vi "Material-Automation-LaunchWirebirdLabsWebsite.vi"(0 "Site to Launch":T1, 11 "error in":errorcluster) -> (15 "error out":errorcluster)   [LabVIEW 2013]
uses:
  Material-Automation-Website.ctl
panel:
  # "Inputs"
  # "Outputs"
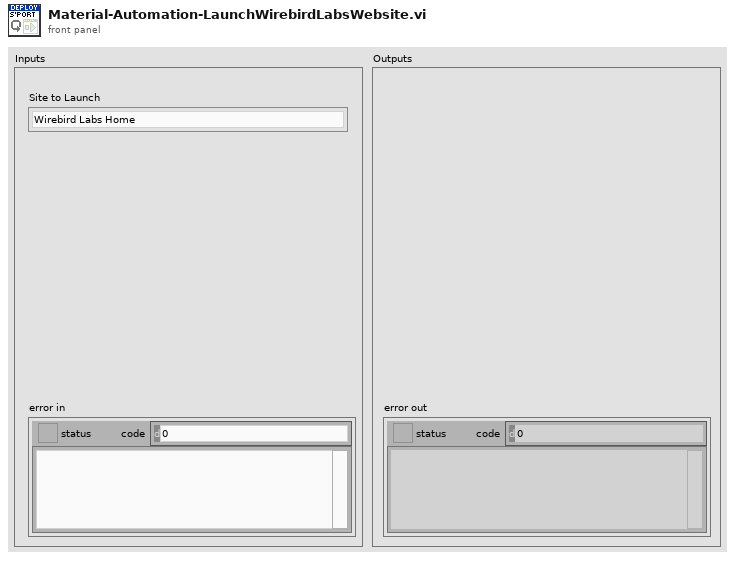
[diagram p1: front panel]
types:
  T1 = typedef "Material-Automation-Website.ctl" = enum16{"Wirebird Labs Home", "Wirebird Labs Support Home", "Wirebird Labs Licensing", "Wirebird Labs Idea Exchange", "Wirebird Labs Report a Bug", "Wirebird Labs Services Status", "Contact Wirebird Labs", "Deploy Documentation", "Deploy Credits", "Deploy Marketing", "Deploy Feature Matrix", "Deploy Purchase", "Deploy Deployment Servers"}
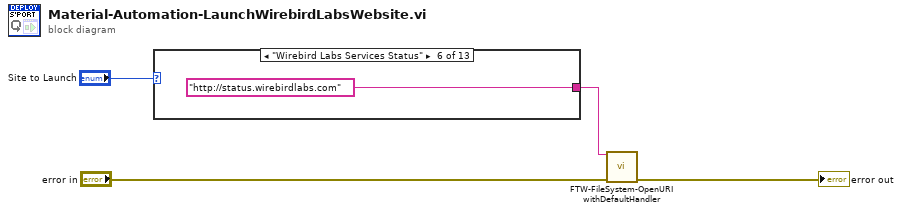
[diagram p0: block diagram]
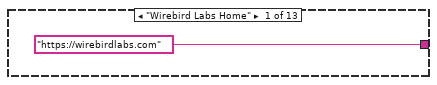
[diagram p2: hidden frame]
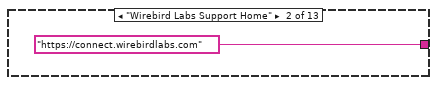
[diagram p3: hidden frame]
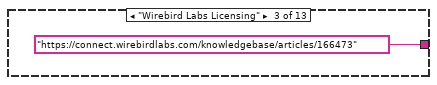
[diagram p4: hidden frame]
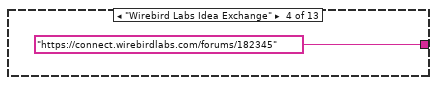
[diagram p5: hidden frame]
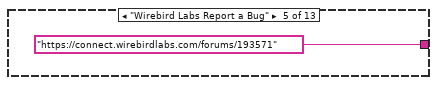
[diagram p6: hidden frame]
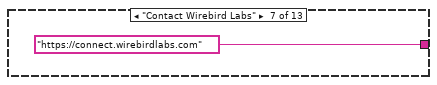
[diagram p7: hidden frame]
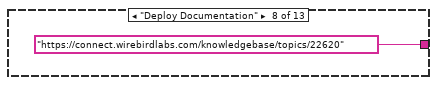
[diagram p8: hidden frame]
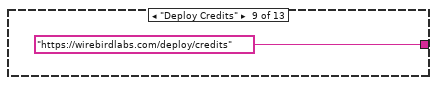
[diagram p9: hidden frame]
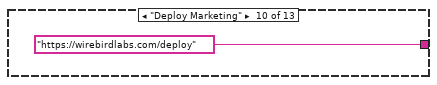
[diagram p10: hidden frame]
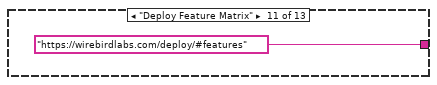
[diagram p11: hidden frame]
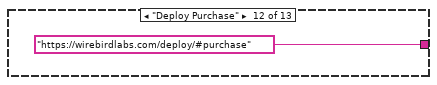
[diagram p12: hidden frame]
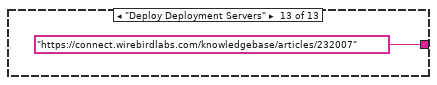
[diagram p13: hidden frame]
diagram:
  n1 = case shown="\"Wirebird Labs Services Status\"" "Site to Launch" {
    tunnel: ["https://wirebirdlabs.com" ("URL") "https://connect.wirebirdlabs.com" ("URL") "https://connect.wirebirdlabs.com/knowledgebase/articles/166473" ("URL") "https://connect.wirebirdlabs.com/forums/182345" ("URL") "https://connect.wirebirdlabs.com/forums/193571" ("URL") "http://status.wirebirdlabs.com" ("URL") "https://connect.wirebirdlabs.com" ("URL") "https://connect.wirebirdlabs.com/knowledgebase/topics/22620" ("URL") "https://wirebirdlabs.com/deploy/credits" ("URL") "https://wirebirdlabs.com/deploy" ("URL") "https://wirebirdlabs.com/deploy/#features" ("URL") "https://wirebirdlabs.com/deploy/#purchase" ("URL") "https://connect.wirebirdlabs.com/knowledgebase/articles/232007" ("URL")] -> w1
    frame "Wirebird Labs Home" {
    }
    frame "Wirebird Labs Support Home" {
    }
    frame "Wirebird Labs Licensing" {
    }
    frame "Wirebird Labs Idea Exchange" {
    }
    frame "Wirebird Labs Report a Bug" {
    }
    frame "Wirebird Labs Services Status" {
    }
    frame "Contact Wirebird Labs" {
    }
    frame "Deploy Documentation" {
    }
    frame "Deploy Credits" {
    }
    frame "Deploy Marketing" {
    }
    frame "Deploy Feature Matrix" {
    }
    frame "Deploy Purchase" {
    }
    frame "Deploy Deployment Servers" {
    }
  }
  n2 = call "FTW-FileSystem-OpenURIwithDefaultHandler.vi"("URI to Open"=w1, "error in"="error in") -> ("error out"=→"error out":errorcluster)  [unwired: 12 in, 1 out]
